vi "Save Xml.vi"(8 "error in":errorcluster caption="错误输入（无错误）", 10 "selected path":path caption="所选路径", 11 "PanelRootNode 输入":refnum<class "PanelRootNode.lvclass"> caption="DNL_LabVIEW Object in") -> (0 "error out":errorcluster caption="错误输出", 3 "PanelRootNode 输出":refnum<class "PanelRootNode.lvclass"> caption="DNL_LabVIEW Object out")   [LabVIEW 2013, in "PanelRootNode.lvclass"]
uses:
  PanelRootNode.lvclass
  <vilib>/xml/Close Reference(Node).vi
  <vilib>/xml/NI_XML.lvlib
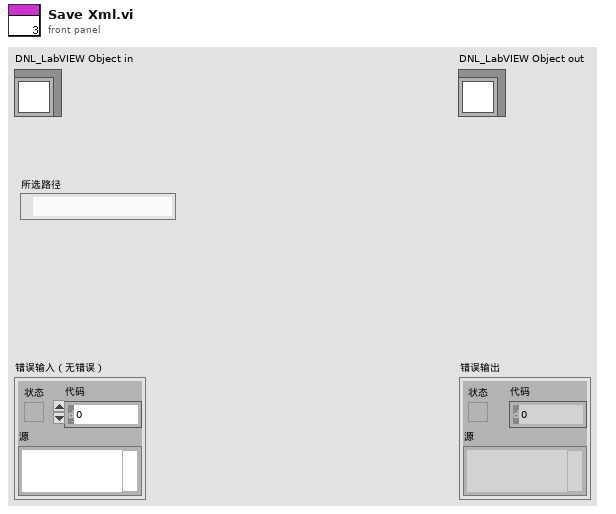
[diagram p1: front panel]
types:
  T1 = cluster{"DOM Ref":refnum<k20>, "Element Ref":refnum<k20>}
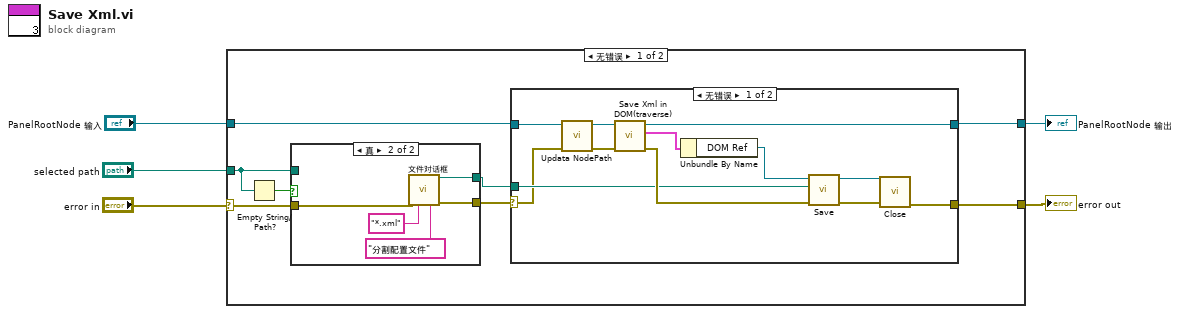
[diagram p0: block diagram]
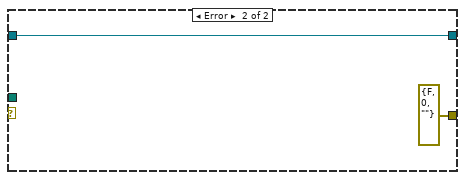
[diagram p3: hidden frame]
diagram:
  n1 = case shown="无错误" "error in" {
    selector: "error in" -> [w9 w36]
    tunnel: [w10 w36] -> w4
    tunnel: [w13 w35] -> w2
    tunnel: "PanelRootNode 输入" -> [w6 w35]
    tunnel: "selected path" -> [w7 _]
    frame No Error {
      n2 = Empty String/Path?(string/path=w7) -> (empty?=w8:bool)
      n3 = case shown="真" w8 {
        tunnel: [w15 w20] -> w12
        tunnel: [w14 w19] -> w11
        tunnel: w9 -> [w14 w18]
        tunnel: w7 -> [w15 _]
        frame False {
        }
        frame True {
          n4 = call "文件对话框"("error in"=w18, "pattern (all files)"="*.xml", "pattern label"="分割配置文件") -> ("selected path"=w20:path, "error out"=w19:errorcluster)  [unwired: 9 in, 2 out]
        }
      }
      n5 = case shown="无错误" w11 {
        selector: w11 -> [w22 _]
        tunnel: w6 -> [w23 w34]
        tunnel: [w32 w34] -> w13
        tunnel: w12 -> [w26 _]
        tunnel: [w25 errorcluster {"status"=FALSE, "code"=0, "source"=""} ("error out")] -> w10
        frame No Error {
          n6 = call-dynamic "Updata NodePath.vi"("error in"=w22, "PanelLinkNode 输入"=w23) -> ("error out"=w21:errorcluster, "PanelLinkNode 输出"=w24:refnum<class "PanelRootNode.lvclass">)  [unwired: 8 in]
          n7 = call "Save Xml in DOM(traverse).vi"("error in"=w21, "PanelRootNode.lvclass"=w24) -> ("error out"=w27:errorcluster, "Data out"=w31:T1, "PanelRootNode out"=w32:refnum<class "PanelRootNode.lvclass">)  [unwired: 7 in]
          n8 = Unbundle By Name(w31) -> ("DOM Ref"=w30:refnum<k20>)
          n9 = call <vilib>:"Save.vi"("error in (no error)"=w27, "XML file path"=w26, "DOM document in"=w30) -> ("error out"=w28:errorcluster, "DOM document out"=w29:refnum<k20>)  [unwired: 6 in, 1 out]
          n10 = call-poly <vilib>:"Close.vi"("error in (no error)"=w28, "node"=w29) -> ("error out"=w25:errorcluster)  [unwired: 7 in]
        }
        frame Error {
        }
      }
    }
    frame Error {
    }
  }
  "error out" <- w4
  "PanelRootNode 输出" <- w2
